vi "QDInstrument_Example.vi"() -> ()   [LabVIEW 2019]
uses:
  <vilib>/Analysis/baseanly.llb/Mean (DBL).vi
  <vilib>/Analysis/NI_AALBase.lvlib
panel:
  in  "Instrument\nType":i32(ring) items=["PPMS", "VersaLab", "DynaCool", "SVSM"]
  in  "Remote":bool=TRUE
  in  "IP Address":string="130.49.180.18"
  out "Field\nStatus":i32(ring) items=["MagnetUnknown"=0, "StablePersistent"=1, "WarmingSwitch"=2, "CoolingSwitch"=3, "StableDriven"=4, "Iterating"=5, "Charging"=6, "Discharging"=7, "CurrentError"=8, "MagnetFailure"=15]
  out "Temperature\nStatus":i32(ring) items=["TemperatureUnknown"=0, "Stable"=1, "Tracking"=2, "Near"=5, "Chasing"=6, "Filling"=7, "Standby"=10, "Disabled"=13, "ImpedanceNotFunction"=14, "TempFailure"=15]
  out "Chamber\nStatus":i32(ring) items=["ChamberUnknown"=0, "PurgedAndSealed"=1, "VentedAndSealed"=2, "Sealed"=3, "Purging"=4, "Venting"=5, "PreHiVac"=6, "HighVac"=7, "PumpContinuous"=8, "VentContinuous"=9, "ChamberFailure"=15]
  out "Field":dbl
  out "Measuring":bool
  in  "Delay":dbl=5.0
  in  "WaitForField":bool=TRUE
  in  "WaitForTemperature":bool=TRUE
  out "Temperature":dbl
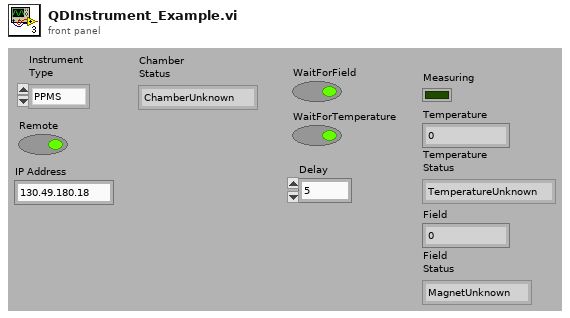
[diagram p1: front panel]
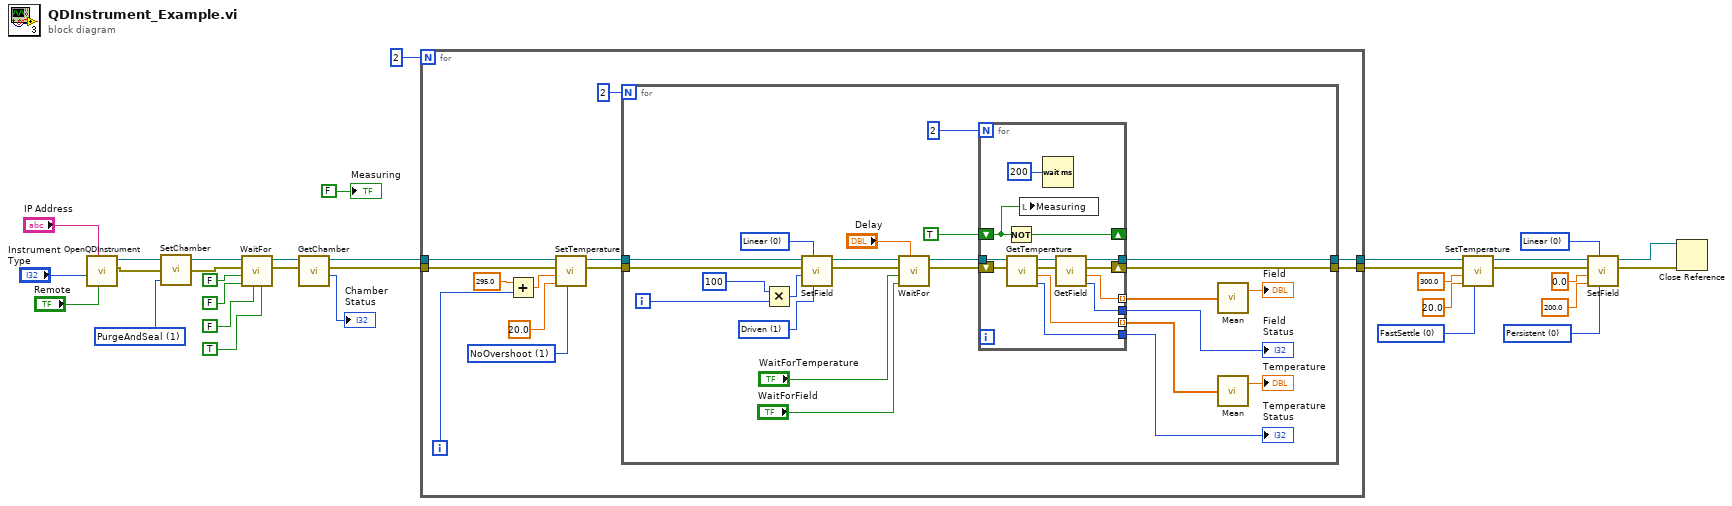
[diagram p0: block diagram]
diagram:
  w2 = 0 items=["Persistent", "Driven"] ("Mode")
  w10 = 0 items=["Linear", "NoOvershoot", "Oscillate"] ("Approach")
  w3 = 0 items=["FastSettle", "NoOvershoot"] ("Approach")
  w14 = 1 items=["Seal", "PurgeAndSeal", "VentAndSeal", "PumpContinuous", "VentContinuous", "HighVacuum"] ("Code")
  n1 = call "OpenQDInstrument.vi"("Remote"="Remote", "IP Address"="IP Address", "Instrument Type"="Instrument\nType") -> ("error out"=w27:errorcluster, "Instrument Ref"=w32:refnum<k24>)  [unwired: 5 in]
  n2 = call "SetChamber.vi"("Code"=w14, "error in (no error)"=w27, "Instrument Ref In"=w32) -> ("error out"=w13:errorcluster, "Instrument Ref Out"=w12:refnum<k24>)  [unwired: 1 out]
  n3 = call "WaitFor.vi"("Wait For Chamber"=TRUE ("WaitForChamber"), "Wait For Position"=FALSE ("WaitForPosition"), "Wait For Field"=FALSE ("WaitForField"), "Wait For Temperature"=FALSE ("WaitForTemperature"), "error in (no error)"=w13, "Instrument Ref In"=w12) -> ("error out"=w28:errorcluster, "Instrument Ref Out"=w25:refnum<k24>)  [unwired: 4 in]
  n4 = call "GetChamber.vi"("error in (no error)"=w28, "Instrument Ref In"=w25) -> ("Chamber\nStatus"=→"Chamber\nStatus":i32, "error out"=w29:errorcluster, "Instrument Ref Out"=w26:refnum<k24>)  [unwired: 2 in, 1 out]
  n5 = for {
    N: 2 -> [_]
    tunnel: w26 -> [w43]
    tunnel: [w38] -> w21
    tunnel: w29 -> [w44]
    tunnel: [w40] -> w23
    i -> [w37]
    w33 = 1 items=["FastSettle", "NoOvershoot"] ("Approach")
    n6 = Add(x=295.0, y=w37) -> (x+y=w35:dbl)
    n7 = call "SetTemperature.vi"("Approach"=w33, "Rate"=20.0, "Temperature"=w35, "error in (no error)"=w44, "Instrument Ref In"=w43) -> ("error out"=w41:errorcluster, "Instrument Ref Out"=w42:refnum<k24>)  [unwired: 2 in, 1 out]
    n8 = for {
      N: 2 -> [_]
      tunnel: w42 -> [w66]
      tunnel: [w63] -> w38
      tunnel: w41 -> [w65]
      tunnel: [w62] -> w40
      i -> [w68]
      w59 = 0 items=["Linear", "NoOvershoot", "Oscillate"] ("Approach")
      w60 = 1 items=["Persistent", "Driven"] ("Mode")
      n9 = Multiply(x=100, y=w68) -> (x*y=w53:i32)
      n10 = call "SetField.vi"("Mode"=w60, "Approach"=w59, "Field"=w53, "error in (no error)"=w65, "Instrument Ref In"=w66) -> ("error out"=w58:errorcluster, "Instrument Ref Out"=w54:refnum<k24>)  [unwired: 2 in, 1 out]
      n11 = call "WaitFor.vi"("Delay"="Delay", "Wait For Field"="WaitForField", "Wait For Temperature"="WaitForTemperature", "error in (no error)"=w58, "Instrument Ref In"=w54) -> ("error out"=w67:errorcluster, "Instrument Ref Out"=w64:refnum<k24>)  [unwired: 5 in]
      n12 = for {
        N: 2 -> [_]
        shift-right: [w81] -> _
        shift-left: TRUE -> [w79]
        shift-right: [w76] -> w62
        shift-left: w67 -> [w78]
        tunnel: w64 -> [w75]
        tunnel: [w73] -> w63
        tunnel: [w70] -> w50
        tunnel: [w69] -> w49
        tunnel: [w71] -> w47 mode=indexing
        tunnel: [w72] -> w48 mode=indexing
        n13 = Not(x=w79) -> (.not. x?=w81:bool)
        n14 = call "GetTemperature.vi"("error in (no error)"=w78, "Instrument Ref In"=w75) -> ("Temperature\nStatus"=w69:i32, "Temperature"=w72:dbl, "error out"=w77:errorcluster, "Instrument Ref Out"=w74:refnum<k24>)  [unwired: 3 in, 1 out]
        n15 = local write "Measuring"(w79) -> ()
        n16 = Wait (ms)(milliseconds to wait=u32 200) -> ()  [unwired: 1 out]
        n17 = call "GetField.vi"("error in (no error)"=w77, "Instrument Ref In"=w74) -> ("Field\nStatus"=w70:i32, "Field"=w71:dbl, "error out"=w76:errorcluster, "Instrument Ref Out"=w73:refnum<k24>)  [unwired: 3 in, 1 out]
      }
      "Field\nStatus" <- w50
      "Temperature\nStatus" <- w49
      n18 = call-poly <vilib>:"Mean.vi"("X"=w47) -> ("mean"=→"Field":dbl)  [unwired: 1 out]
      n19 = call-poly <vilib>:"Mean.vi"("X"=w48) -> ("mean"=→"Temperature":dbl)  [unwired: 1 out]
    }
  }
  n20 = call "SetTemperature.vi"("Approach"=w3, "Rate"=20.0, "Temperature"=300.0, "error in (no error)"=w23, "Instrument Ref In"=w21) -> ("error out"=w7:errorcluster, "Instrument Ref Out"=w6:refnum<k24>)  [unwired: 2 in, 1 out]
  n21 = call "SetField.vi"("Mode"=w2, "Approach"=w10, "Rate"=200.0, "Field"=0.0, "error in (no error)"=w7, "Instrument Ref In"=w6) -> ("error out"=w31:errorcluster, "Instrument Ref Out"=w30:refnum<k24>)  [unwired: 1 in, 1 out]
  n22 = Close Reference(reference=w30, error in (no error)=w31) -> ()  [unwired: 1 out]
  "Measuring" <- FALSE
